vi "正常显示强装十六进制显示1.vi"(1 "正常格式显示字符串":string) -> (0 "十六进制格式显示":string)   [LabVIEW 2016, in "数据传输系统.lvlib" / "自动更新.lvlib" / "TCP文件传输系统.lvlib" / "TCP发送文件.lvlib"]
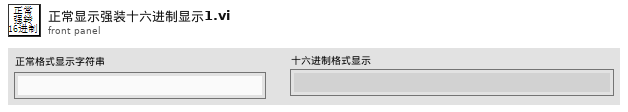
[diagram p1: front panel]
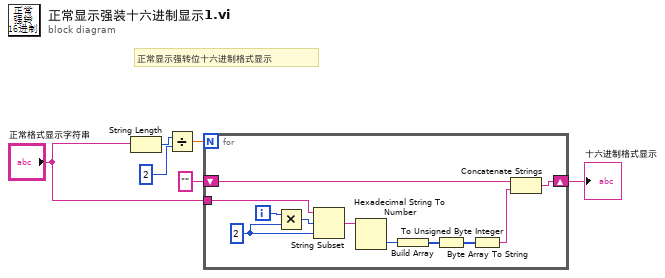
[diagram p0: block diagram]
diagram:
  # "正常显示强转位十六进制格式显示"
  n1 = String Length(string="正常格式显示字符串") -> (length=w6:i32)
  n2 = Divide(x=w6, y=2) -> (x/y=w3:dbl)
  n3 = for {
    N: w3 -> [_]
    shift-right: [w10] -> w2
    shift-left: "" -> [w11]
    tunnel: "正常格式显示字符串" -> [w14]
    i -> [w17]
    w15 = 2 ("y")
    n4 = Multiply(x=w17, y=w15) -> (x*y=w16:i32)
    n5 = String Subset(string=w14, offset (0)=w16, length (rest)=w15) -> (substring=w13:string)
    n6 = Hexadecimal String To Number(string=w13) -> (number=w8:u32)  [unwired: 2 in, 1 out]
    n7 = Build Array(w8) -> (w7:u32[])
    n8 = To Unsigned Byte Integer(number=w7) -> (unsigned 8bit integer=w9:u8[])
    n9 = Byte Array To String(unsigned byte array=w9) -> (string=w12:string)
    n10 = Concatenate Strings(w11, w12) -> (w10:string)
  }
  "十六进制格式显示" <- w2
